vi "Set Sub Panel Coins.vi"(8 "error in (no error)":errorcluster, 10 "Sub Panel Coins":refnum<vi>, 11 "MXN Actor in":refnum<class "MXN Actor.lvclass">) -> (0 "error out":errorcluster, 3 "MXN Actor out":refnum<class "MXN Actor.lvclass">)   [LabVIEW 2020, in "MXN Actor.lvlib" / "MXN Actor.lvclass"]
uses:
  MXN Actor.lvclass
  MXN Actor.lvclass/MXN Actor.ctl
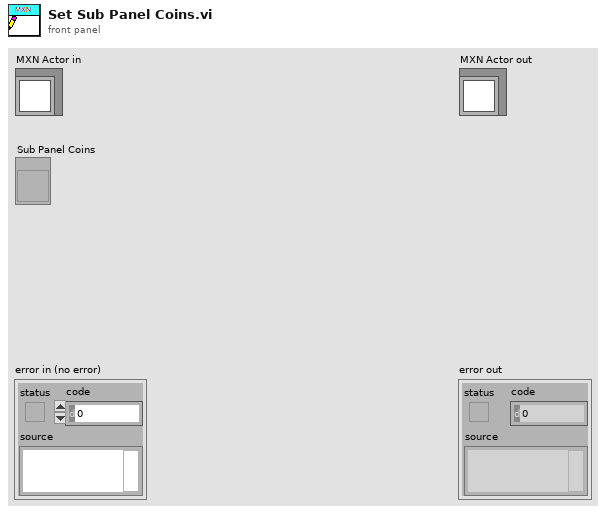
[diagram p1: front panel]
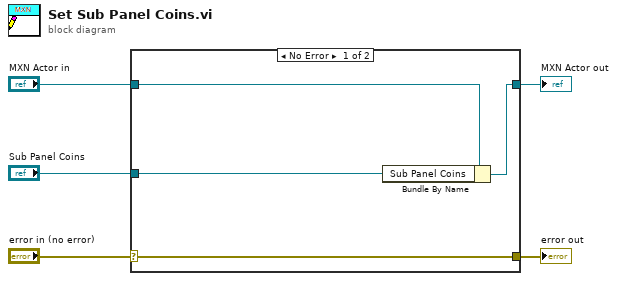
[diagram p0: block diagram]
diagram:
  n1 = case shown="No Error" "error in (no error)" {
    selector: "error in (no error)" -> [w9 w10]
    tunnel: [w9 w10] -> w4
    tunnel: [w7 w11] -> w2
    tunnel: "MXN Actor in" -> [w8 w11]
    tunnel: "Sub Panel Coins" -> [w6 _]
    frame No Error {
      n2 = Bundle By Name(cluster=w8, "Sub Panel Coins"=w6) -> (w7:refnum<class "MXN Actor.lvclass">)
    }
    frame Error {
    }
  }
  "error out" <- w4
  "MXN Actor out" <- w2
